vi "Build_Asylum_GetLabel.vi"(8 "error in (no error)":errorcluster, 11 "parameterName":string) -> (0 "error out":errorcluster, 3 "Command":string)   [LabVIEW 2016]
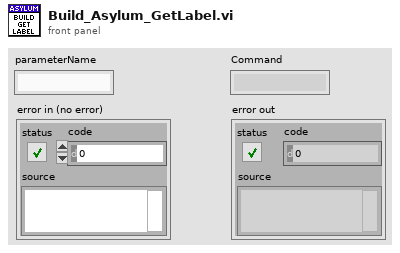
[diagram p1: front panel]
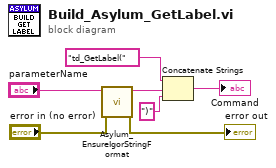
[diagram p0: block diagram]
diagram:
  n1 = call "Asylum_EnsureIgorStringFormat.vi"("error in (no error)"="error in (no error)", "Value"="parameterName") -> ("error out"=→"error out":errorcluster, "Value"=w3:string)  [unwired: 8 in]
  n2 = Concatenate Strings("td_GetLabel(", w3, ")" ("string")) -> (→"Command":string)
